vi "GEA2 Initialize.vi"(0 "Board Index":i32, 5 "Source Address":u8=228 format="%.0x", 11 "error in":errorcluster) -> (4 "GEA2 Reference Out":refnum<k24>, 8 "Board ID":string, 15 "error out":errorcluster)   [LabVIEW 2016, in "GEA2_Toolkit.lvlib"]
doc: "This VI uses .NET DLLs to initialize a GEA2 connection over USB. The output is a reference to the newly opened GEA2 connection."
uses:
  library/GEA2_Toolkit.lvlib
  C:/TechnologyLab/NI-2010/Trunk/Utility/LabVIEW GEA2 Toolkit v1.0.0.0/Appliance.NET/GeaCommunication.dll
  Appliance.NET/GeaCommunication.dll
  C:/TechnologyLab/NI-2010/Trunk/Utility/LabVIEW GEA2 Toolkit v1.0.0.0/Appliance.NET/GeaCommunication.Usb.dll
  Appliance.NET/GeaCommunication.Usb.dll
panel:
  out "Running":bool
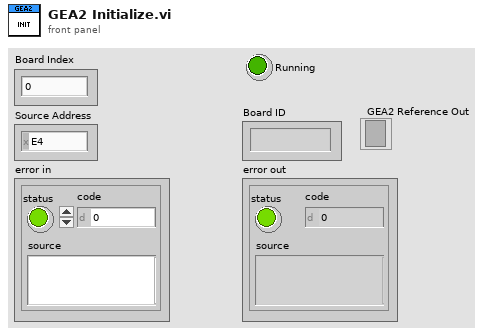
[diagram p1: front panel]
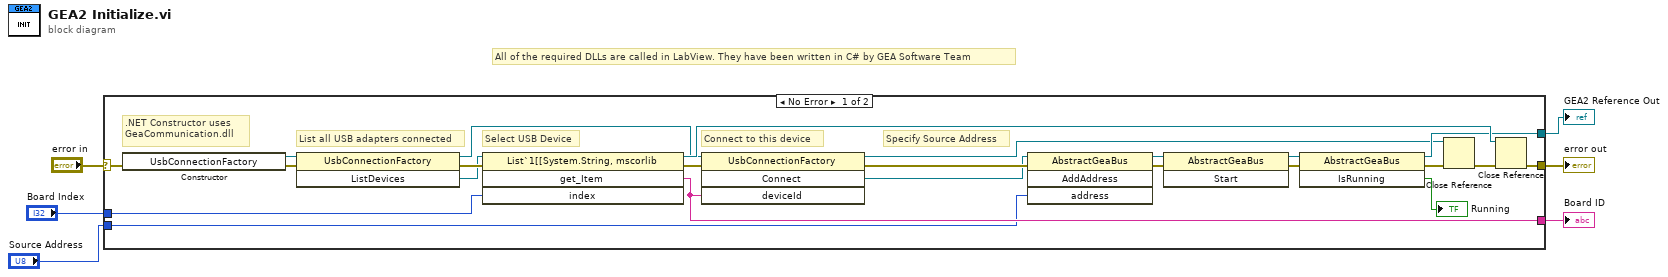
[diagram p0: block diagram]
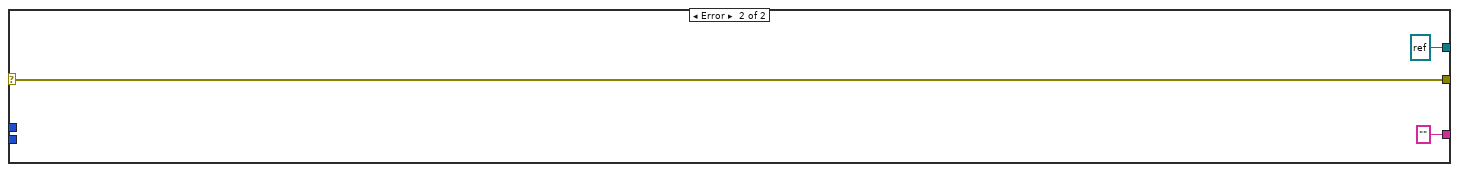
[diagram p2: hidden frame]
diagram:
  # "All of the required DLLs are called in LabView. They have been written in C# by GEA Software Team"
  n1 = case shown="No Error" "error in" {
    selector: "error in" -> [w27 w32]
    tunnel: "Board Index" -> [w28 _]
    tunnel: [w23 w32] -> w6
    tunnel: [w9 refnum<k24> refnum ("Connect")] -> w1
    tunnel: "Source Address" -> [w16 _]
    tunnel: [w19 "" ("get_Item")] -> w2
    frame No Error {
      # "Specify Source Address"
      # "Connect to this device"
      # "Select USB Device"
      # "List all USB adapters connected"
      # ".NET Constructor uses\nGeaCommunication.dll"
      n2 = constructor class="UsbConnectionFactory"(error in=w27) -> (reference out=w22:refnum<k24>, error out=w26:errorcluster)  [unwired: 2 in, 1 out]
      n3 = invoke class="UsbConnectionFactory" method="ListDevices"(reference=w22, error in=w26) -> (reference out=w20:refnum<k24>, error out=w29:errorcluster, "ListDevices"=w21:refnum<k24>)  [unwired: 1 in]
      n4 = invoke class="List`1[[System.String, mscorlib" method="get_Item"(reference=w21, error in=w29, "index"=w28) -> (reference out=w25:refnum<k24>, error out=w18:errorcluster, "get_Item"=w19:string)  [unwired: 1 in, 1 out]
      n5 = invoke class="UsbConnectionFactory" method="Connect"(reference=w20, error in=w18, "deviceId"=w19) -> (reference out=w8:refnum<k24>, error out=w17:errorcluster, "Connect"=w7:refnum<k24>)  [unwired: 1 in, 1 out]
      n6 = invoke class="AbstractGeaBus" method="AddAddress"(reference=w7, error in=w17, "address"=w16) -> (reference out=w14:refnum<k24>, error out=w15:errorcluster)  [unwired: 1 in, 2 out]
      n7 = invoke class="AbstractGeaBus" method="Start"(reference=w14, error in=w15) -> (reference out=w13:refnum<k24>, error out=w12:errorcluster)  [unwired: 1 in, 1 out]
      n8 = invoke class="AbstractGeaBus" method="IsRunning"(reference=w13, error in=w12) -> (reference out=w9:refnum<k24>, error out=w10:errorcluster, "IsRunning"=→"Running":bool)  [unwired: 1 in]
      n9 = Close Reference(reference=w8, error in (no error)=w10) -> (error out=w24:errorcluster)
      n10 = Close Reference(reference=w25, error in (no error)=w24) -> (error out=w23:errorcluster)
    }
    frame Error {
    }
  }
  "error out" <- w6
  "Board ID" <- w2
  "GEA2 Reference Out" <- w1
